vi "Update_Install_Path.vi"(8 "error in (no error)":errorcluster, 10 "destName":string, 11 "userLabel in":refnum<class "userLabel.lvclass">) -> (0 "error out":errorcluster, 3 "userLabel out":refnum<class "userLabel.lvclass">)   [LabVIEW 2020, in "userLabel.lvclass"]
uses:
  <vilib>/AppBuilder/IB_Classes/Destination/userLabel/userLabel.lvclass
  <vilib>/AppBuilder/IB_Classes/Destination/userLabel/userLabel.lvclass/userLabel.ctl
  <vilib>/AppBuilder/IB_Classes/Destination/IB_Destination.lvclass
  e:/builds/penguin/labview/branches/2020/dev/dist/vi.lib/AppBuilder/IB_Classes/Destination/IB_Destination.lvclass
  e:/builds/penguin/labview/branches/2020/dev/dist/vi.lib/AppBuilder/IB_Classes/Destination/userLabel/userLabel.lvclass
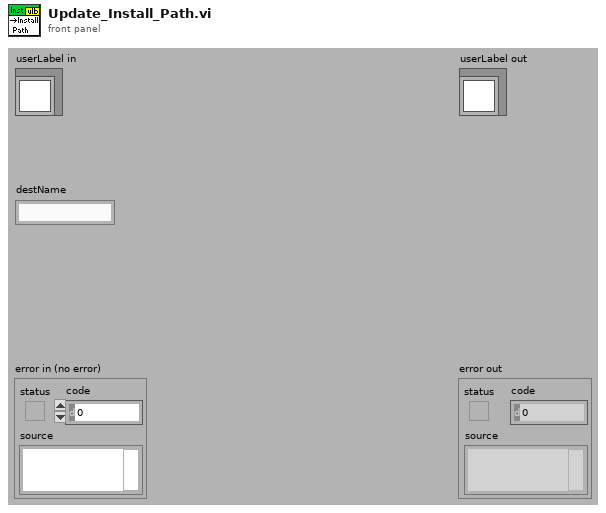
[diagram p1: front panel]
types:
  T1 = typedef "IB_Destination.ctl" = cluster{"name":string, "unlock":bool, "parentTag":string, "destTag":string, "eng_installPath":string}
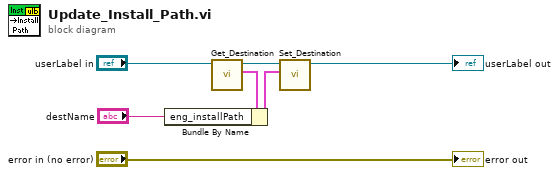
[diagram p0: block diagram]
diagram:
  n1 = call <vilib>:"Get_Destination.vi"("IB_Destination in"="userLabel in") -> ("data"=w5:T1, "IB_Destination out"=w6:refnum<class "userLabel.lvclass">)  [unwired: 1 in, 8 out]
  n2 = Bundle By Name(cluster=w5, "eng_installPath"="destName") -> (w4:T1)
  n3 = call <vilib>:"Set_Destination.vi"("data"=w4, "IB_Destination in"=w6) -> ("IB_Destination out"=→"userLabel out":refnum<class "userLabel.lvclass">)  [unwired: 1 in, 8 out]
  "error out" <- "error in (no error)"
